vi "Excel Set Excel Location.vi"(1 "column":i32, 2 "row":i32) -> (0 "cell's name":string)   [LabVIEW 2010, in "NI_ReportGenerationToolkit.lvlib"]
doc: "Returns the Excel syntax name of a cell that you identify by row and column indexes."
uses:
  <vilib>/addons/_office/NI_ReportGenerationToolkit.lvlib
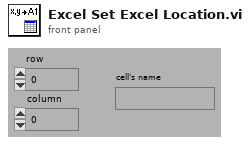
[diagram p1: front panel]
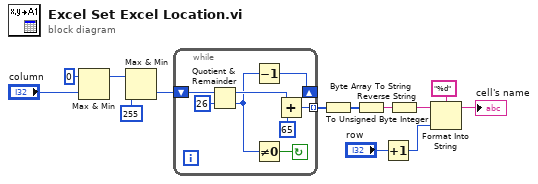
[diagram p0: block diagram]
diagram:
  n1 = Max & Min(x=0, y="column") -> (max(x,y)=w5:i32)  [unwired: 1 out]
  n2 = Max & Min(x=w5, y=255) -> (min(x,y)=w4:i32)  [unwired: 1 out]
  n3 = while {
    tunnel: [w18] -> w10 mode=indexing
    shift-left: w4 -> [w20]
    shift-right: [w14] -> _
    stop <- w19 continue-if-true
    n4 = Quotient & Remainder(x=w20, y=26) -> (x-y*floor(x/y)=w16:i32, floor(x/y)=w15:i32)
    n5 = Decrement(x=w15) -> (x-1=w14:i32)
    n6 = Not Equal To 0?(x=w15) -> (x != 0?=w19:bool)
    n7 = Add(x=w16, y=65) -> (x+y=w18:i32)
  }
  n8 = To Unsigned Byte Integer(number=w10) -> (unsigned 8bit integer=w9:u8[])
  n9 = Byte Array To String(unsigned byte array=w9) -> (string=w8:string)
  n10 = Increment(x="row") -> (x+1=w1:i32)
  n11 = Reverse String(1:w8) -> (0:w7:string)
  n12 = Format Into String(format string="%d" ("Format String"), initial string=w7, w1) -> (resulting string=→"cell's name":string)  [unwired: 1 in, 1 out]
